vi "Observe Data.vi"(6 "Time Stamp":timestamp, 8 "error in (no error)":errorcluster, 9 "Value":variant, 10 "Datum Name":string, 11 "ExampleSimpleRootModel in":refnum<class "SimpleRootModel.lvclass">) -> (0 "error out":errorcluster, 3 "ExampleSimpleRootModel out":refnum<class "SimpleRootModel.lvclass">)   [LabVIEW 2018, in "MVAExamples.lvlib" / "SimpleRootModel.lvclass"]
doc: "<License>\nCopyright © 2017 Composed Systems, LLC | All rights reserved\nwww.composed.io\n\nAuthor: Ethan Stern <ethan.stern@composed.io>\n\nThis software is provided \"AS IS\" WITHOUT WARRANTIES, either express or implied, AND IS FOR EDUCATIONAL PURPOSES ONLY.\n</License>"
uses:
  SimpleRootModel.lvclass
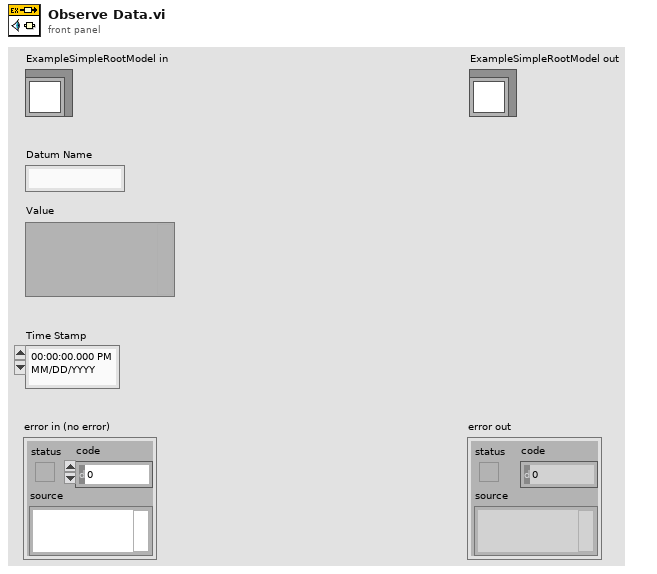
[diagram p1: front panel]
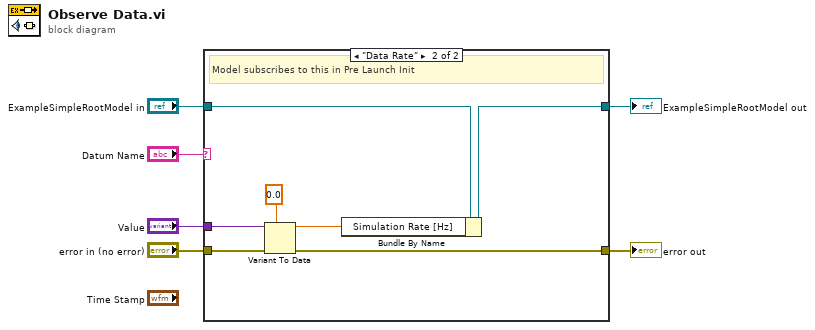
[diagram p0: block diagram]
diagram:
  n1 = case shown="\"Data Rate\"" "Datum Name" {
    tunnel: "ExampleSimpleRootModel in" -> [w8 w15]
    tunnel: "error in (no error)" -> [w7 w13]
    tunnel: [w8 w14] -> w3
    tunnel: [w7 w12] -> w2
    tunnel: "Value" -> [_ w11]
    frame Default {
    }
    frame "Data Rate" {
      # "Model subscribes to this in Pre Launch Init"
      n2 = Variant To Data(error in=w13, type=0.0, Variant=w11) -> (data=w9:dbl, error out=w12:errorcluster)
      n3 = Bundle By Name(cluster=w15, "Simulation Rate [Hz]"=w9) -> (w14:refnum<class "SimpleRootModel.lvclass">)
    }
  }
  "error out" <- w2
  "ExampleSimpleRootModel out" <- w3
